vi "Write TCPServer.vi"(8 "error in (no error)":errorcluster, 10 "TCPServer.lvclass":refnum<class "TCPServer.lvclass">, 11 "MonoCommunicator in":refnum<class "MonoCommunicator.lvclass">) -> (0 "error out":errorcluster, 3 "MonoCommunicator out":refnum<class "MonoCommunicator.lvclass">)   [LabVIEW 2016, in "MonoCommunicator.lvclass"]
uses:
  MonoCommunicator.lvclass
  ts_labview_tcp/TCPServer/TCPServer.lvclass
  MonoCommunicator.lvclass/MonoCommunicator.ctl
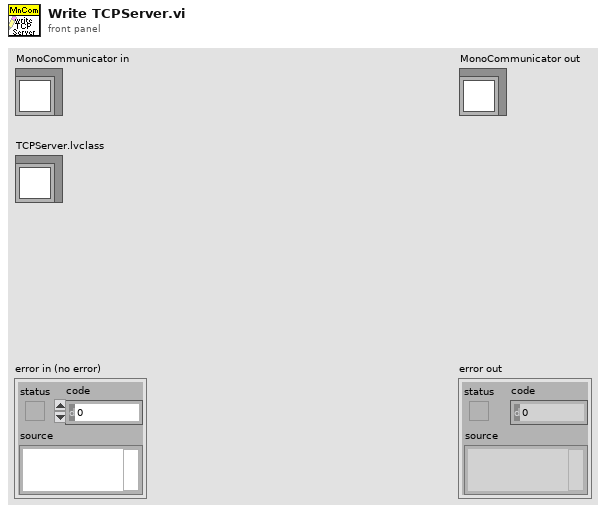
[diagram p1: front panel]
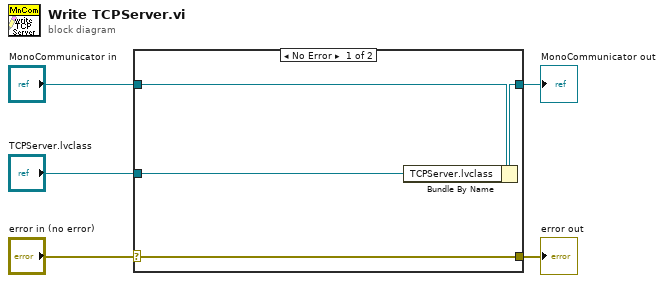
[diagram p0: block diagram]
diagram:
  n1 = case shown="No Error" "error in (no error)" {
    selector: "error in (no error)" -> [w9 w10]
    tunnel: [w9 w10] -> w4
    tunnel: [w7 w11] -> w2
    tunnel: "MonoCommunicator in" -> [w8 w11]
    tunnel: "TCPServer.lvclass" -> [w6 _]
    frame No Error {
      n2 = Bundle By Name(cluster=w8, "TCPServer.lvclass"=w6) -> (w7:refnum<class "MonoCommunicator.lvclass">)
    }
    frame Error {
    }
  }
  "error out" <- w4
  "MonoCommunicator out" <- w2
